vi "DrawRec两条竖直线.vi"(9 "Color":u32(colorbox)=16711680, 10 "Rectangle":T3, 11 "Image":T2) -> (1 "起始和终止线":T1={"起始线"={"P1"={"X1"=3212.0, "Y1"=2837.0}, "P2"={"X2"=3212.0, "Y2"=2872.0}}, "终止线"={"P1"={"X1"=3243.0, "Y1"=2837.0}, "P2"={"X2"=3243.0, "Y2"=2872.0}}}, 3 "Image Out":T2)   [LabVIEW 2014]
uses:
  <vilib>/vision/Image Controls.llb/IMAQ Image.ctl
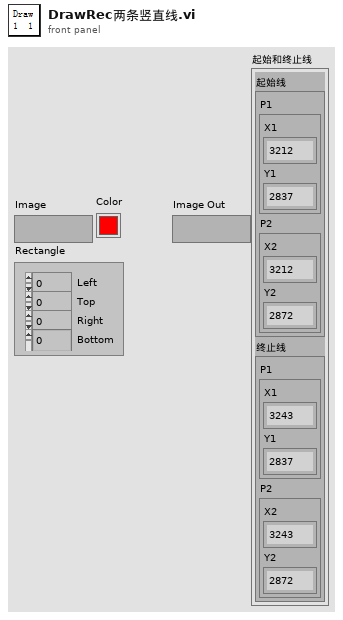
[diagram p1: front panel]
types:
  T1 = cluster{"起始线":cluster{"P1":cluster{"X1":dbl, "Y1":dbl}, "P2":cluster{"X2":dbl, "Y2":dbl}}, "终止线":cluster{"P1":cluster{"X1":dbl, "Y1":dbl}, "P2":cluster{"X2":dbl, "Y2":dbl}}}
  T2 = typedef "IMAQ Image.ctl" = refnum<image>
  T3 = cluster{"Left":i32, "Top":i32, "Right":i32, "Bottom":i32}
  T4 = cluster{cluster{"Right":i32, "Top":i32}, cluster{"Right":i32, "Bottom":i32}}
  T5 = cluster{cluster{"Left":i32, "Top":i32}, cluster{"Left":i32, "Bottom":i32}}
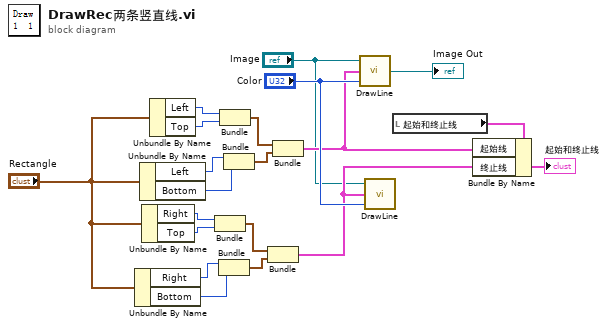
[diagram p0: block diagram]
diagram:
  n1 = Unbundle By Name("Rectangle") -> ("Right"=w11:i32, "Bottom"=w12:i32)
  n2 = Unbundle By Name("Rectangle") -> ("Left"=w18:i32, "Bottom"=w17:i32)
  n3 = Unbundle By Name("Rectangle") -> ("Right"=w9:i32, "Top"=w10:i32)
  n4 = Unbundle By Name("Rectangle") -> ("Left"=w20:i32, "Top"=w19:i32)
  n5 = Bundle("Right"=w9, "Top"=w10) -> (w13:cluster{"Right":i32, "Top":i32})  [unwired: 1 in]
  n6 = Bundle("Right"=w11, "Bottom"=w12) -> (w14:cluster{"Right":i32, "Bottom":i32})  [unwired: 1 in]
  n7 = Bundle("Left"=w20, "Top"=w19) -> (w16:cluster{"Left":i32, "Top":i32})  [unwired: 1 in]
  n8 = Bundle("Left"=w18, "Bottom"=w17) -> (w15:cluster{"Left":i32, "Bottom":i32})  [unwired: 1 in]
  n9 = Bundle(w13, w14) -> (w2:T4)  [unwired: 1 in]
  n10 = Bundle(w16, w15) -> (w5:T5)  [unwired: 1 in]
  n11 = call "DrawLine.vi"("Color"="Color", "Edge Points"=w5, "img in"="Image") -> ("Image Out"=→"Image Out":T2)
  n12 = call "DrawLine.vi"("Color"="Color", "Edge Points"=w2, "img in"="Image") -> ()  [unwired: 1 out]
  n13 = local read "起始和终止线"() -> (w3:T1)
  n14 = Bundle By Name(cluster=w3, "起始线"=w5, "终止线"=w2) -> (→"起始和终止线":T1)
